vi "Defer Message Until Cleaned Up.vi"(9 "Tracked Actor Count":i32, 10 "IModel in":refnum<class "IModel.lvclass">, 11 "Message in":refnum<class "Message.lvclass">) -> (2 "IModel out":refnum<class "IModel.lvclass">)   [LabVIEW 2017, in "IModel.lvlib" / "IModel.lvclass"]
uses:
  <vilib>/gpm_packages/@cs/mva-core/Source/IModel/IModel/IModel.lvclass
  C:/Program Files/National Instruments/LabVIEW 2017/vi.lib/gpm_packages/@cs/mva-core/Source/IObserver/IObserver/IObserver.lvclass
  <vilib>/ActorFramework/Message/Message.lvclass
  <vilib>/gpm_packages/@cs/mva-core/Source/IModel/IModel/IModel.lvclass/IModel.ctl
  <vilib>/gpm_packages/@cs/mva-core/Source/IObserver/IObserver/IObserver.lvclass/IObserver.ctl
  <vilib>/gpm_packages/@cs/event-logger/Source/Composed Log/LoggerReference/LoggerReference.lvclass/LoggerReference.ctl
  <vilib>/gpm_packages/@cs/event-logger/Source/Composed Log/LoggerReference/Log Event.vi
  <vilib>/gpm_packages/@cs/event-logger/Source/Composed Log/LoggerReference/Log.vi
  <vilib>/gpm_packages/@cs/event-logger/Source/Composed Log/LoggerReference/Get Valid Event Time.vi
  <vilib>/gpm_packages/@cs/event-logger/Source/Composed Log/LoggerReference/Remove Stale Logs.vi
  <vilib>/gpm_packages/@cs/mva-core/Source/IObserver/IObserver/IObserver.lvclass
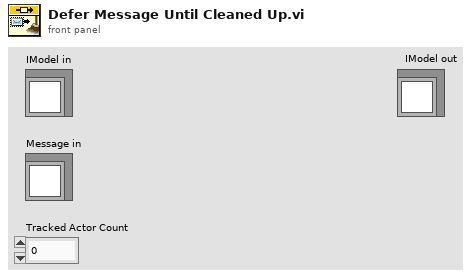
[diagram p1: front panel]
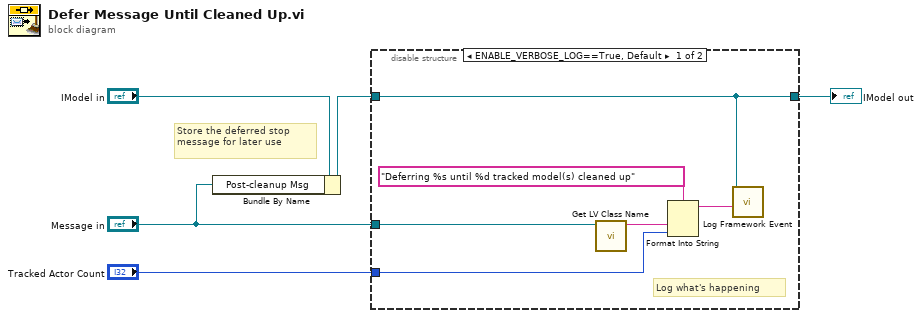
[diagram p0: block diagram]
diagram:
  # "Store the deferred stop\nmessage for later use"
  n1 = Bundle By Name(cluster="IModel in", "Post-cleanup Msg"="Message in") -> (w2:refnum<class "IModel.lvclass">)
  n2 = disable-structure shown="ENABLE_VERBOSE_LOG==True, Default" {
    disable-tunnel: "Message in" -> [w11 _]
    disable-tunnel: "Tracked Actor Count" -> [w7 _]
    disable-tunnel: w2 -> [w6 w12]
    disable-tunnel: [w6 w12] -> w1
    frame condition #0 (active) {
      # "Log what's happening"
      n3 = call <vilib>:"Get LV Class Name.vi"("object"=w11) -> ("class name"=w8:string)  [unwired: 9 in, 1 out]
      n4 = Format Into String(format string="Deferring %s until %d tracked model(s) cleaned up", w8, w7) -> (resulting string=w9:string)  [unwired: 2 in, 1 out]
      n5 = call <vilib>:"Log Framework Event.vi"("Data To Log"=w9, "IObserver in"=w6) -> ()  [unwired: 9 in, 1 out]
    }
    frame condition #1 {
    }
  }
  "IModel out" <- w1
